vi "Update Control Names in VIs.vi"(6 "Build Folder":path, 8 "error in (no error)":errorcluster, 10 "New Name":string, 11 "VI Reference":refnum<vi>) -> (0 "error out":errorcluster, 3 "vi ref out":refnum<vi>)   [LabVIEW 2020, in "ADAS_IO_Template_MDO.lvclass"]
uses:
  ADAS_IO_Template_MDO.lvclass
  ADAS_IO_Template_MDO.lvclass/ADAS_IO_Template_MDO.ctl
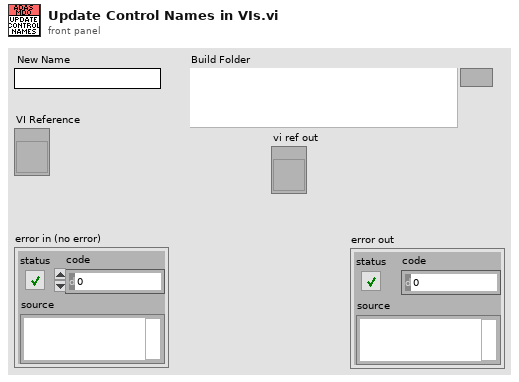
[diagram p1: front panel]
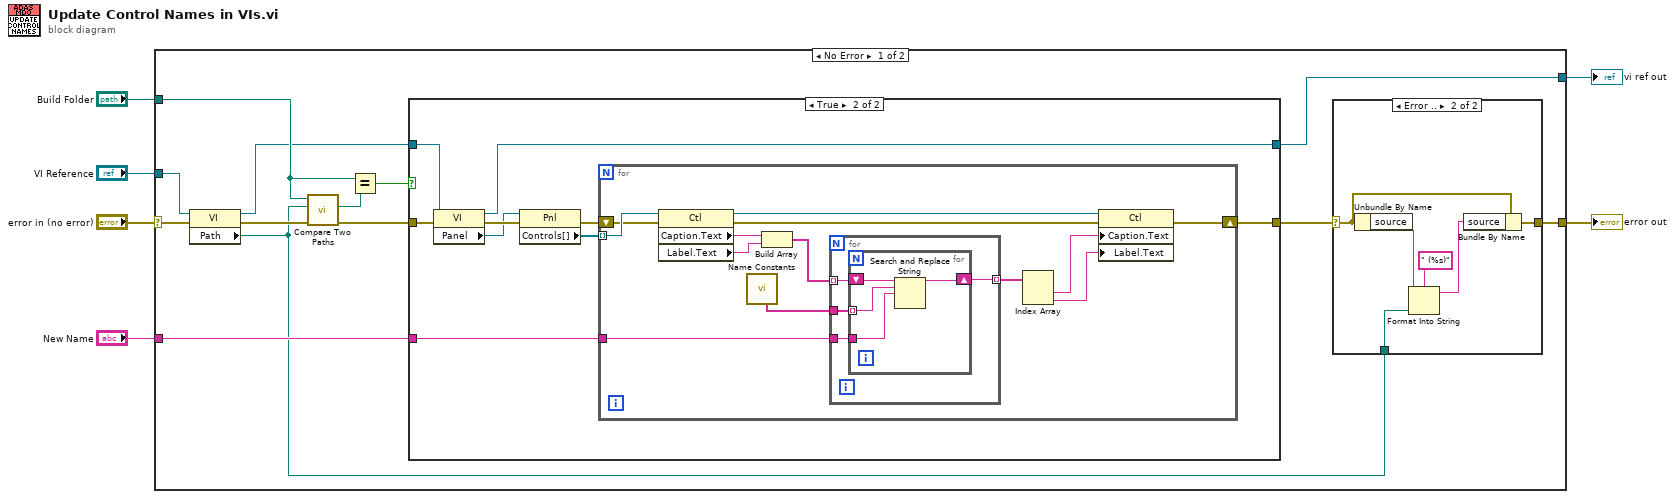
[diagram p0: block diagram]
diagram:
  n1 = case shown="No Error" "error in (no error)" {
    selector: "error in (no error)" -> [w17 w60]
    tunnel: "VI Reference" -> [w19 w59]
    tunnel: "New Name" -> [w18 _]
    tunnel: [w15 w60] -> w4
    tunnel: "Build Folder" -> [w11 _]
    tunnel: [w7 w59] -> w1
    frame No Error {
      n2 = property class="VI"(reference=w19, error in=w17) -> (reference out=w8:refnum<vi>, error out=w14:errorcluster, "Path"=w9:path)
      n3 = call <vilib>:"Compare Two Paths.vi"("error in (no error)"=w14, "Path 2"=w9, "Path 1"=w11) -> ("error out"=w13:errorcluster, "Common Path"=w12:path)  [unwired: 5 in, 2 out]
      n4 = Equal?(x=w11, y=w12) -> (x = y?=w10:bool)
      n5 = case shown="True" w10 {
        tunnel: w13 -> [w21 w26]
        tunnel: w18 -> [_ w28]
        tunnel: [w21 w27] -> w16
        tunnel: w8 -> [w20 w23]
        tunnel: [w20 w22] -> w7
        frame False {
        }
        frame True {
          n6 = property class="VI"(reference=w23, error in=w26) -> (reference out=w22:refnum<vi>, error out=w25:errorcluster, "Panel"=w24:refnum<vi>)
          n7 = property class="Pnl"(reference=w24, error in=w25) -> (error out=w29:errorcluster, "Controls[]"=w30:refnum<vi>[])  [unwired: 1 out]
          n8 = for {
            tunnel: w30 -> [w43] mode=indexing
            shift-right: [w35] -> w27
            shift-left: w29 -> [w41]
            tunnel: w28 -> [w34]
            n9 = property class="Ctl"(reference=w43, error in=w41) -> (reference out=w42:refnum<vi>, error out=w36:errorcluster, "Caption.Text"=w40:string, "Label.Text"=w39:string)
            n10 = call "Name Constants.vi"() -> ("Strings to Replace w Name"=w37:string[])  [unwired: 9 in, 2 out]
            n11 = Build Array(w40, w39) -> (w38:string[])
            n12 = for {
              tunnel: w38 -> [w47] mode=indexing
              tunnel: w37 -> [w46]
              tunnel: w34 -> [w45]
              tunnel: [w44] -> w33 mode=indexing
              n13 = for {
                tunnel: w46 -> [w50] mode=indexing
                tunnel: w45 -> [w49]
                shift-right: [w48] -> w44
                shift-left: w47 -> [w51]
                n14 = Search and Replace String(input string=w51, search string=w50, replace string=w49) -> (result string=w48:string)  [unwired: 5 in, 3 out]
              }
            }
            n15 = Index Array(array=w33) -> (element #1=w32:string, element #2=w31:string)  [unwired: 2 in]
            n16 = property class="Ctl"(reference=w42, error in=w36, "Caption.Text"=w32, "Label.Text"=w31) -> (error out=w35:errorcluster)  [unwired: 1 out]
          }
        }
      }
      n17 = case shown="Error .." w16 {
        selector: w16 -> [w52 w58]
        tunnel: [w52 w57] -> w15
        tunnel: w9 -> [_ w53]
        frame No Error {
        }
        frame Error {
          n18 = Unbundle By Name(w58) -> ("source"=w56:string)
          n19 = Format Into String(format string=" (%s)", initial string=w56, w53) -> (resulting string=w54:string)  [unwired: 1 in, 1 out]
          n20 = Bundle By Name(cluster=w58, "source"=w54) -> (w57:errorcluster)
        }
      }
    }
    frame Error {
    }
  }
  "error out" <- w4
  "vi ref out" <- w1
